vi "Clear.vi"(11 "Priority Queue in":refnum<class "NI_Robotics_Priority Queue.lvclass">) -> (1 "nElements":i32, 2 "Open List":T1[](array[typedef]), 3 "Priority Queue out":refnum<class "NI_Robotics_Priority Queue.lvclass">)   [LabVIEW 2017, in "NI_Robotics_Priority Queue.lvclass"]
uses:
  <vilib>/robotics/Navigation/shared/Priority Queue/NI_Robotics_Priority Queue.lvclass
  <vilib>/robotics/Navigation/shared/Priority Queue/Open List Element.ctl
  <vilib>/robotics/Navigation/shared/MapNode/AbstractMapNode/NI_Robotics_AbstractMapNode.lvclass
  <vilib>/robotics/Navigation/shared/Priority Queue/NI_Robotics_Priority Queue.lvclass/NI_Robotics_Priority Queue.ctl
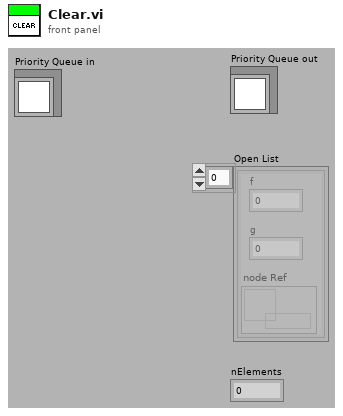
[diagram p1: front panel]
types:
  T1 = typedef "NI_Robotics_Priority Queue.lvclass/Open List Element.ctl" = cluster{"f":dbl, "g":dbl, "node Ref":refnum<data-value>}
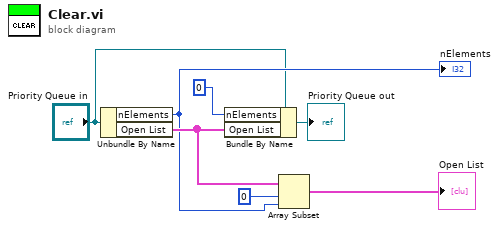
[diagram p0: block diagram]
diagram:
  n1 = Unbundle By Name("Priority Queue in") -> ("nElements"=w2:i32, "Open List"=w5:T1[])
  "nElements" <- w2
  n2 = Bundle By Name(cluster="Priority Queue in", "nElements"=0, "Open List"=w5) -> (→"Priority Queue out":refnum<class "NI_Robotics_Priority Queue.lvclass">)
  n3 = Array Subset(array=w5, index=0, length=w2) -> (→"Open List":T1[])
